vi "Get Library Refnum.vi"(11 "error in":errorcluster) -> (4 "library refnum":refnum<vi>, 6 "project refnum":refnum<vi>, 15 "error out":errorcluster)   [LabVIEW 2021, in "Converter.lvlib"]
uses:
  Converter.lvlib
  Converter Reusables/Converter Reusables.lvlib
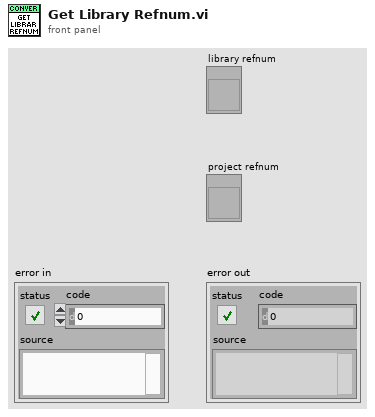
[diagram p1: front panel]
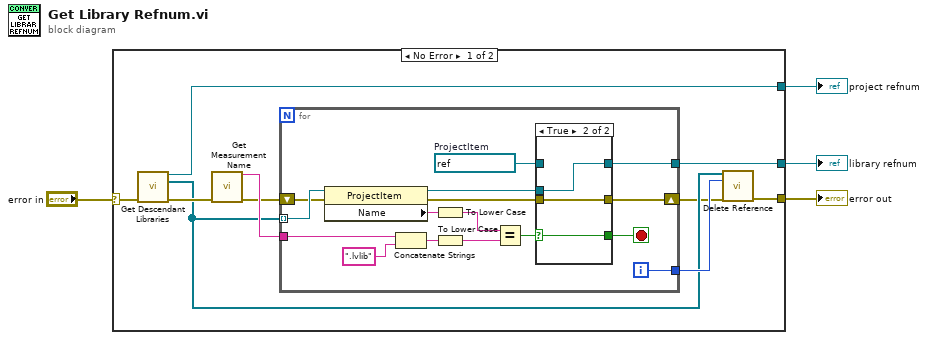
[diagram p0: block diagram]
diagram:
  n1 = case shown="No Error" "error in" {
    selector: "error in" -> [w12 w37]
    tunnel: [w14 _] -> w4
    tunnel: [w6 w37] -> w3
    tunnel: [w13 _] -> w2
    frame No Error {
      n2 = call "Get Descendant Libraries.vi"("error in"=w12) -> ("project out"=w13:refnum<vi>, "all descendents"=w7:refnum<vi>[], "error out"=w10:errorcluster)  [unwired: 12 in]
      n3 = call "Get Measurement Name.vi"("error in"=w10) -> ("name out"=w11:string, "error out"=w9:errorcluster)  [unwired: 13 in]
      n4 = for {
        tunnel: w7 -> [w30] mode=indexing
        tunnel: [w24] -> w14
        tunnel: w11 -> [w23]
        tunnel: [w17] -> w8
        shift-right: [w15] -> w5
        shift-left: w9 -> [w22]
        i -> [w17]
        stop <- w25 stop-if-true
        w28 = refnum<vi> refnum  # ProjectItem
        n5 = property class="ProjectItem"(reference=w30, error in=w22) -> (reference out=w27:refnum<vi>, error out=w26:errorcluster, "Name"=w29:string)
        n6 = Concatenate Strings(w23, ".lvlib" ("string")) -> (w21:string)
        n7 = To Lower Case(string=w29) -> (all lower case string=w19:string)
        n8 = To Lower Case(string=w21) -> (all lower case string=w18:string)
        n9 = Equal?(x=w19, y=w18) -> (x = y?=w16:bool)
        n10 = case shown="True" w16 {
          selector: w16 -> [w32 w35]
          tunnel: w27 -> [_ w36]
          tunnel: [w31 w34] -> w15
          tunnel: [w33 w36] -> w24
          tunnel: w28 -> [w33 _]
          tunnel: [w32 w35] -> w25
          tunnel: w26 -> [w31 w34]
          frame False {
          }
          frame True {
          }
        }
      }
      n11 = call "Delete Reference.vi"("all descendents"=w7, "numeric"=w8, "error in"=w5) -> ("error out"=w6:errorcluster)  [unwired: 12 in]
    }
    frame Error {
    }
  }
  "library refnum" <- w4
  "error out" <- w3
  "project refnum" <- w2
